vi "dfd_FXPSimu AccSub (vector).vi"(5 "quantize output?":bool, 7 "FXP OP":T4={"source"=0, "is floating?"=FALSE, "o-mode"=enum."Wrap", "q-mode"=enum."Nearest", "signed?"=FALSE, "fwl"=0, "high limit"=0.0, "low limit"=0.0, "full range"=0.0} {"source" items=["Coef a/k"=0, "Coef b/v"=7, "Input"=1, "Output"=2, "Multiplicand"=3, "Product"=4, "Sum"=5, "Delay"=6, "Gain"=8]}, 8 "filtering statistics in":T3(array[cluster]) {"statistics information"."min value" format="%.2f"; "statistics information"."max value" format="%.2f"; "Quantizer Source" items=["Coefficients a/k"=0, "Coefficients b/v"=7, "Input"=1, "Output"=2, "Multiplicand"=3, "Product"=4, "Sum"=5, "Delay"=6]}, 10 "addends":ext[](array[numeric]) format="%.2f", 11 "acc in":ext format="%.2f") -> (0 "filtering statistics out":T3(array[cluster]) {"statistics information"."min value" format="%.2f"; "statistics information"."max value" format="%.2f"; "Quantizer Source" items=["Coefficients a/k"=0, "Coefficients b/v"=7, "Input"=1, "Output"=2, "Multiplicand"=3, "Product"=4, "Sum"=5, "Delay"=6]}, 3 "acc out":ext format="%.2f")   [LabVIEW 2017, in "NI_DigFilter_FXP.lvlib"]
uses:
  <vilib>/addons/Digital Filter Design/NI_DigFilter_FXP.lvlib
  <vilib>/addons/Digital Filter Design/_Objects.llb/dfd_FXP Operation.ctl
  <vilib>/addons/Digital Filter Design/_Objects.llb/dfd_Internal Quantization Srcs.ctl
  <vilib>/addons/Digital Filter Design/_Objects.llb/DFD Quantization Sources.ctl
  <vilib>/addons/Digital Filter Design/_Objects.llb/DFD FXP Statistics Data.ctl
  <vilib>/addons/Digital Filter Design/NI_DigFilterLicensed.lvlib
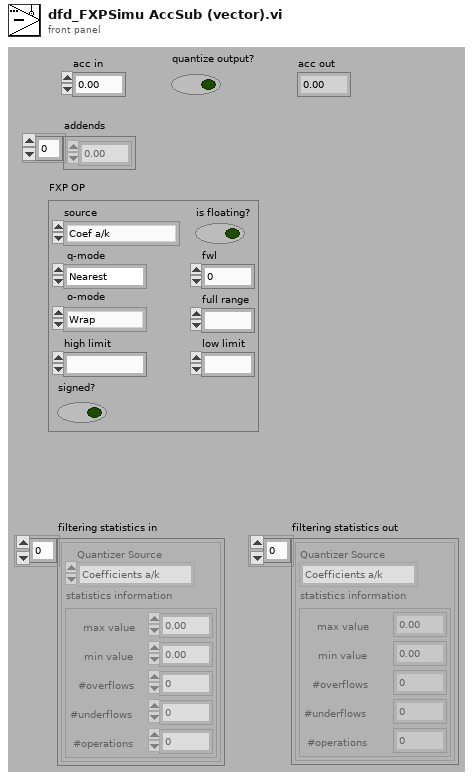
[diagram p1: front panel]
types:
  T1 = typedef "NI_DigFilterLicensed.lvlib/DFD Quantization Sources.ctl" = u16
  T2 = typedef "NI_DigFilterLicensed.lvlib/DFD FXP Statistics Data.ctl" = cluster{"max value":ext, "min value":ext, "#overflows":i32, "#underflows":i32, "#operations":i32}
  T3 = cluster{"Quantizer Source":T1, "statistics information":T2}[]
  T4 = typedef "dfd_FXP Operation.ctl" = cluster{"source":T5, "is floating?":bool, "o-mode":enum16{"Saturation", "Wrap"}, "q-mode":enum16{"Nearest", "Truncation"}, "signed?":bool, "fwl":i16, "high limit":ext, "low limit":ext, "full range":ext}
  T5 = typedef "NI_DigFilterLicensed.lvlib/dfd_Internal Quantization Srcs.ctl" = u16
  T6 = cluster{"Quantizer Source":T1, "statistics information":T2}
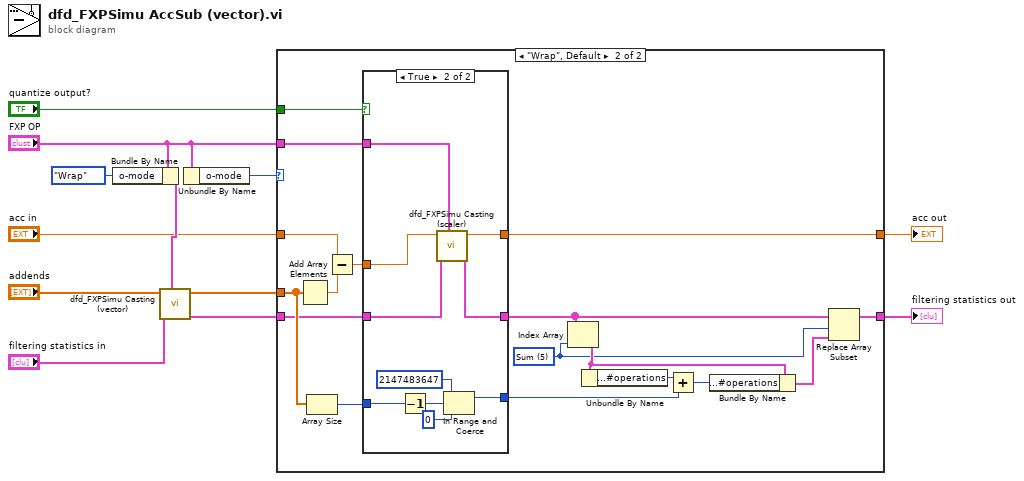
[diagram p0: block diagram]
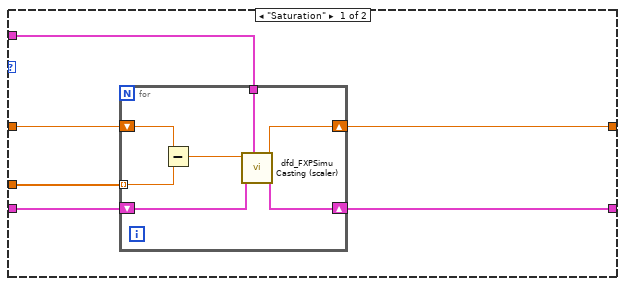
[diagram p2: hidden frame]
diagram:
  n1 = Bundle By Name(cluster="FXP OP", "o-mode"=enum16{"Saturation", "Wrap"}."Wrap" ("o_mode")) -> (w8:T4)
  n2 = call <vilib>:"dfd_FXPSimu Casting (vector).vi"("FXP op"=w8, "filtering statistics in"="filtering statistics in", "values in"="addends") -> ("filtering statistics out"=w7:T3, "values out"=w1:ext[])  [unwired: 7 out]
  n3 = Unbundle By Name("FXP OP") -> ("o-mode"=w5:enum16{"Saturation", "Wrap"})
  n4 = case shown="\"Wrap\", Default" w5 {
    tunnel: [w13 w37] -> w12
    tunnel: [w14 w26] -> w10
    tunnel: w7 -> [w18 w36]
    tunnel: "quantize output?" -> [_ w38]
    tunnel: "FXP OP" -> [w17 w34]
    tunnel: "acc in" -> [w16 w42]
    tunnel: w1 -> [w15 w40]
    frame "Saturation" {
      n5 = for {
        tunnel: w17 -> [w24]
        shift-right: [w20] -> w14
        shift-left: w18 -> [w25]
        tunnel: w15 -> [w22] mode=indexing
        shift-right: [w19] -> w13
        shift-left: w16 -> [w23]
        n6 = Subtract(x=w23, y=w22) -> (x-y=w21:ext)
        n7 = call <vilib>:"dfd_FXPSimu Casting (scaler).vi"("FXP op"=w24, "filtering statistics in"=w25, "value in"=w21) -> ("filtering statistics out"=w20:T3, "value out"=w19:ext)  [unwired: 7 out]
      }
    }
    frame "Wrap", Default {
      w27 = T5 5 items=["Coef a/k"=0, "Coef b/v"=7, "Input"=1, "Output"=2, "Multiplicand"=3, "Product"=4, "Sum"=5, "Delay"=6, "Gain"=8] ("source")
      n8 = Add Array Elements(numeric array=w40) -> (sum=w41:ext)
      n9 = Array Size(array=w40) -> (size(s)=w35:i32)
      n10 = Subtract(x=w42, y=w41) -> (x-y=w39:ext)
      n11 = case shown="True" w38 {
        tunnel: w39 -> [w45 w55]
        tunnel: w34 -> [_ w54]
        tunnel: [w45 w53] -> w37
        tunnel: w36 -> [w44 w52]
        tunnel: [w44 w51] -> w30
        tunnel: w35 -> [w43 w50]
        tunnel: [w43 w46] -> w32
        frame False {
        }
        frame True {
          n12 = Decrement(x=w50) -> (x-1=w49:i32)
          n13 = call <vilib>:"dfd_FXPSimu Casting (scaler).vi"("FXP op"=w54, "filtering statistics in"=w52, "value in"=w55) -> ("filtering statistics out"=w51:T3, "value out"=w53:ext)  [unwired: 7 out]
          n14 = In Range and Coerce(upper limit=2147483647, x=w49, lower limit=0) -> (coerced(x)=w46:i32)  [unwired: 1 out]
        }
      }
      n15 = Index Array(array=w30, index=w27) -> (element=w29:T6)
      n16 = Unbundle By Name(w29) -> ("statistics information.#operations"=w33:i32)
      n17 = Add(x=w33, y=w32) -> (x+y=w28:i32)
      n18 = Bundle By Name(cluster=w29, "statistics information.#operations"=w28) -> (w31:T6)
      n19 = Replace Array Subset(array=w30, new element=w31, index=w27) -> (w26:T3)
    }
  }
  "acc out" <- w12
  "filtering statistics out" <- w10
